vi "device_set_timeout.vi"(8 "error in (no error)":errorcluster, 10 "Значение параметра":sgl=15.0, 11 "paramUnicorn in":T1={"conParam"={"ReadIntParam"=FALSE, "ReadDescrParam"=FALSE, "ReadFloatParam"=FALSE, "debug"=FALSE, "ReadJSON"=FALSE, "IP_address"="", "N_attempts"=0, "type_con"=enum."Serial", "MB_address"=0, "VISA"="", "connection ID"=refnum, "nameDevices"="", "timeout"=0, "port"=0, "type_version"="", "baud_rate"=0, "VersionControl"=FALSE, "TCP_conn"=FALSE, "WindowSize"=700}, "Param"={"NumParam"={"NTelem"=0, "NInt"=0, "NFloat"=0, "NTable"=0}, "ParamInt"=[], "Telemetry"=[], "Table"=[], "ParamFloat"=[]}}) -> (0 "error IO":errorcluster, 3 "ParamOut":T1={"conParam"={"ReadIntParam"=TRUE, "ReadDescrParam"=FALSE, "ReadFloatParam"=TRUE, "debug"=FALSE, "ReadJSON"=TRUE, "IP_address"="192.168.1.216", "N_attempts"=3, "type_con"=enum."TCP", "MB_address"=1, "VISA"="COM1", "connection ID"=refnum, "nameDevices"="", "timeout"=3000, "port"=2000, "type_version"="0F0C0001", "baud_rate"=115200, "VersionControl"=TRUE, "TCP_conn"=TRUE, "WindowSize"=700}, "Param"={"NumParam"={"NTelem"=201, "NInt"=16, "NFloat"=10, "NTable"=2}, "ParamInt"=[{"ID"="Режим работы", "Num"=0, "Name"="", "Type"="", "Enum"="", "Desc"="", "Unit"="", "Access"="", "FormatStr"="", "Min"=0, "Max"=0}, {"ID"="", "Num"=0, "Name"="", "Type"="", "Enum"="", "Desc"="", "Unit"="", "Access"="", "FormatStr"="", "Min"=0, "Max"=0}, {"ID"="", "Num"=0, "Name"="", "Type"="", "Enum"="", "Desc"="", "Unit"="", "Access"="", "FormatStr"="", "Min"=0, "Max"=0}, {"ID"="", "Num"=0, "Name"="", "Type"="", "Enum"="", "Desc"="", "Unit"="", "Access"="", "FormatStr"="", "Min"=0, "Max"=0}, {"ID"="", "Num"=0, "Name"="", "Type"="", "Enum"="", "Desc"="", "Unit"="", "Access"="", "FormatStr"="", "Min"=0, "Max"=0}, {"ID"="", "Num"=0, "Name"="", "Type"="", "Enum"="", "Desc"="", "Unit"="", "Access"="", "FormatStr"="", "Min"=0, "Max"=0}, {"ID"="ModeWork", "Num"=0, "Name"="", "Type"="", "Enum"="", "Desc"="", "Unit"="", "Access"="", "FormatStr"="", "Min"=0, "Max"=0}], "Telemetry"=[], "Table"=[], "ParamFloat"=[]}})   [LabVIEW 2017]
uses:
  Unicorn Labview Library/Control/unicorn_Param.ctl
  Unicorn Labview Library/Control/unicorn_conn.ctl
  Unicorn Labview Library/Control/unicorn_JSON.ctl
  Unicorn Labview Library/Control/unicorn_ParamInt.ctl
  Unicorn Labview Library/Control/unicorn_Telemetry.ctl
  Unicorn Labview Library/Control/unicorn_Table.ctl
  Unicorn Labview Library/Control/unicorn_ParamFloat.ctl
  Unicorn Labview Library/Unicorn Library.lvlib
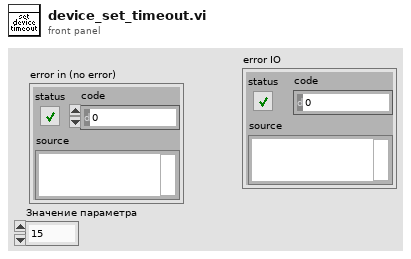
[diagram p1: front panel]
types:
  T1 = typedef "Unicorn Library.lvlib/unicorn_Param.ctl" = cluster{"conParam":T2, "Param":T3}
  T2 = typedef "Unicorn Library.lvlib/unicorn_conn.ctl" = cluster{"ReadIntParam":bool, "ReadDescrParam":bool, "ReadFloatParam":bool, "debug":bool, "ReadJSON":bool, "IP_address":string, "N_attempts":i32, "type_con":enum16{"Serial", "TCP"}, "MB_address":i32, "VISA":refnum<visa-resource-name>, "connection ID":refnum<k5>, "nameDevices":string, "timeout":i32, "port":u16, "type_version":string, "baud_rate":u32, "VersionControl":bool, "TCP_conn":bool, "WindowSize":i32}
  T3 = typedef "Unicorn Library.lvlib/unicorn_JSON.ctl" = cluster{"NumParam":cluster{"NTelem":i32, "NInt":i32, "NFloat":i32, "NTable":i32}, "ParamInt":T4, "Telemetry":T5, "Table":T6, "ParamFloat":T7}
  T4 = typedef "Unicorn Library.lvlib/unicorn_ParamInt.ctl" = cluster{"ID":string, "Num":i32, "Name":string, "Type":string, "Enum":string, "Desc":string, "Unit":string, "Access":string, "FormatStr":string, "Min":i32, "Max":i32}[]
  T5 = typedef "Unicorn Library.lvlib/unicorn_Telemetry.ctl" = cluster{"ID":string, "Num":i32, "Name":string, "Desc":string, "Unit":string, "FormatStr":string, "Min":i32, "Max":i32}[]
  T6 = typedef "Unicorn Library.lvlib/unicorn_Table.ctl" = cluster{"Num":i32, "Access":string, "ColumnCount":i32, "NeedParamPrepare":bool, "Columns":cluster{"Column":i32, "Desc":string, "Name":string}[], "DataType":string, "FormatStr":string, "ID":string, "Name":string, "RowCount":i32, "Rows":cluster{"Desc":string, "ID":string, "Max":i32, "Min":i32, "Name":string, "Row":i32, "Unit":string}[], "Type":string}[]
  T7 = typedef "Unicorn Library.lvlib/unicorn_ParamFloat.ctl" = cluster{"ID":string, "Num":i32, "Name":string, "Type":string, "Enum":string, "Desc":string, "Unit":string, "Access":string, "FormatStr":string, "Min":i32, "Max":i32}[]
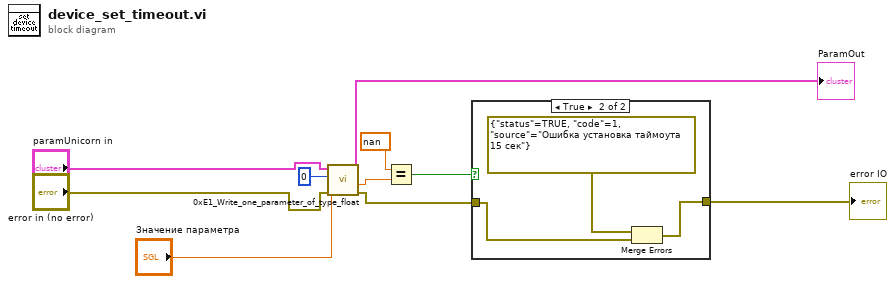
[diagram p0: block diagram]
diagram:
  n1 = call "0xE1_Write_one_parameter_of_type_float.vi"("error in"="error in (no error)", "Значение параметра"="Значение параметра", "Номер параметра"=0, "ParamIn"="paramUnicorn in") -> ("error out"=w10:errorcluster, "Значение параметра 2"=w7:sgl, "ParamOut"=→"ParamOut":T1)  [unwired: 4 in, 1 out]
  n2 = Equal?(x=sgl nan, y=w7) -> (x = y?=w9:bool)
  n3 = case shown="True" w9 {
    tunnel: w10 -> [w11 w13]
    tunnel: [w11 w12] -> w1
    frame False {
    }
    frame True {
      n4 = Merge Errors(errorcluster {"status"=TRUE, "code"=1, "source"="Ошибка установка таймоута 15 сек"} ("error constant"), w13) -> (w12:errorcluster)
    }
  }
  "error IO" <- w1
